vi "writeBits.vi"(0 "I2C Ref Out":T3, 5 "Params":T2={"length"=0, "bitStart"=0, "data"=0, "Register Addresses"=107} {"Register Addresses" items=["SELF_TEST_X"=13, "SELF_TEST_Y"=14, "SELF_TEST_Z"=15, "SELF_TEST_A"=16, "SMPLRT_DIV"=25, "CONFIG"=26, "GYRO_CONFIG"=27, "ACCEL_CONFIG"=28, "MOT_THR"=31, "FIFO_EN"=35, "I2C_MST_CTRL"=36, "I2C_SLV0_ADDR"=37, "I2C_SLV0_REG"=38, "I2C_SLV0_CTRL"=39, "I2C_SLV1_ADDR"=40, "I2C_SLV1_REG"=41, "I2C_SLV1_CTRL"=42, "I2C_SLV2_ADDR"=43, "I2C_SLV2_REG"=44, "I2C_SLV2_CTRL"=45, "I2C_SLV3_ADDR"=46, "I2C_SLV3_REG"=47, "I2C_SLV3_CTRL"=48, "I2C_SLV4_ADDR"=49, "I2C_SLV4_REG"=50, "I2C_SLV4_DO"=51, "I2C_SLV4_CTRL"=52, "I2C_SLV4_DI"=53, "I2C_MST_STATUS"=54, "INT_PIN_CFG"=55, "INT_ENABLE"=56, "INT_STATUS"=58, "ACCEL_XOUT_H"=59, "ACCEL_XOUT_L"=60, "ACCEL_YOUT_H"=61, "ACCEL_YOUT_L"=62, "ACCEL_ZOUT_H"=63, "ACCEL_ZOUT_L"=64, "TEMP_OUT_H"=65, "TEMP_OUT_L"=66, "GYRO_XOUT_H"=67, "GYRO_XOUT_L"=68, "GYRO_YOUT_H"=69, "GYRO_YOUT_L"=70, "GYRO_ZOUT_H"=71, "GYRO_ZOUT_L"=72, "EXT_SENS_DATA_00"=73, "EXT_SENS_DATA_01"=74, "EXT_SENS_DATA_02"=75, "EXT_SENS_DATA_03"=76, "EXT_SENS_DATA_04"=77, "EXT_SENS_DATA_05"=78, "EXT_SENS_DATA_06"=79, "EXT_SENS_DATA_07"=80, "EXT_SENS_DATA_08"=81, "EXT_SENS_DATA_09"=82, "EXT_SENS_DATA_10"=83, "EXT_SENS_DATA_11"=84, "EXT_SENS_DATA_12"=85, "EXT_SENS_DATA_13"=86, "EXT_SENS_DATA_14"=87, "EXT_SENS_DATA_15"=88, "EXT_SENS_DATA_16"=89, "EXT_SENS_DATA_17"=90, "EXT_SENS_DATA_18"=91, "EXT_SENS_DATA_19"=92, "EXT_SENS_DATA_20"=93, "EXT_SENS_DATA_21"=94, "EXT_SENS_DATA_22"=95, "EXT_SENS_DATA_23"=96, "I2C_SLV0_DO"=99, "I2C_SLV1_DO"=100, "I2C_SLV2_DO"=101, "I2C_SLV3_DO"=102, "I2C_MST_DELAY_CTRL"=103, "SIGNAL_PATH_RESET"=104, "MOT_DETECT_CTRL"=105, "USER_CTRL"=106, "PWR_MGMT_1"=107, "PWR_MGMT_2"=108, "FIFO_COUNTH"=114, "FIFO_COUNTL"=115, "FIFO_R_W"=116, "WHO_AM_I"=117]}, 11 "error in (no error)":errorcluster) -> (4 "I2C Ref Out 2":T3={"myRIO Reference"={"myRIO Model"=enum."Unknown", "myRIO Hardware Reference"={"Generic FPGA Reference"=refnum, "Allow multiple opens"=FALSE}}, "I2C Channels Enum"=enum."Not Connected", "I2C Configuration"={"I2C Transfer Rate"=enum."Fast mode (400 kbps)"}}, 15 "error out":errorcluster)   [LabVIEW 2016]
uses:
  <vilib>/myRIO/Instrument Drivers/Onboard IO/I2C/typedefs/I2C Reference.ctl
  <vilib>/myRIO/Common/Instrument Driver Framework/Utilities/typedefs/myRIO Generic Hardware Reference.ctl
  <vilib>/myRIO/Common/Instrument Driver Framework/Utilities/typedefs/Hardware Version Enum.ctl
  <vilib>/myRIO/Common/Instrument Driver Framework/Utilities/typedefs/myRIO v1.0 Reference.ctl
  <vilib>/myRIO/Common/Instrument Driver Framework/Utilities/typedefs/Generic FPGA Reference.ctl
  <vilib>/myRIO/Common/Instrument Driver Framework/myRIO v1.0/I2C/typedefs/I2C Channels Enum.ctl
  <vilib>/myRIO/Instrument Drivers/Onboard IO/I2C/typedefs/I2C Configuration.ctl
  <vilib>/myRIO/Instrument Drivers/Onboard IO/I2C/typedefs/I2C Transfer Rate.ctl
  LIFA MPU-60X0 LV9/RegisterAddresses.ctl
  LIFA MPU-60X0 LV9/DeviceAddresses.ctl
  <vilib>/myRIO/Common/Instrument Driver Framework/myRIO v1.0/I2C/vis/myRIO v1.0 Write I2C.vi
  <vilib>/myRIO/Common/Instrument Driver Framework/myRIO v1.0/I2C/vis/myRIO v1.0 Read I2C.vi
  <vilib>/myRIO/Common/Instrument Driver Framework/roboRIO v1.0/I2C/vis/roboRIO v1.0 Write I2C.vi
  <vilib>/myRIO/Common/Instrument Driver Framework/roboRIO v1.0/I2C/vis/roboRIO v1.0 Read I2C.vi
  <vilib>/Utility/error.llb/Error Cluster From Error Code.vi
  <vilib>/myRIO/Instrument Drivers/Onboard IO/I2C/I2C.lvlib
  LIFA MPU-60X0 LV9/LIFA MPU-60X0.lvlib
panel:
  out "x .or. y?":u8
  out "element":u8
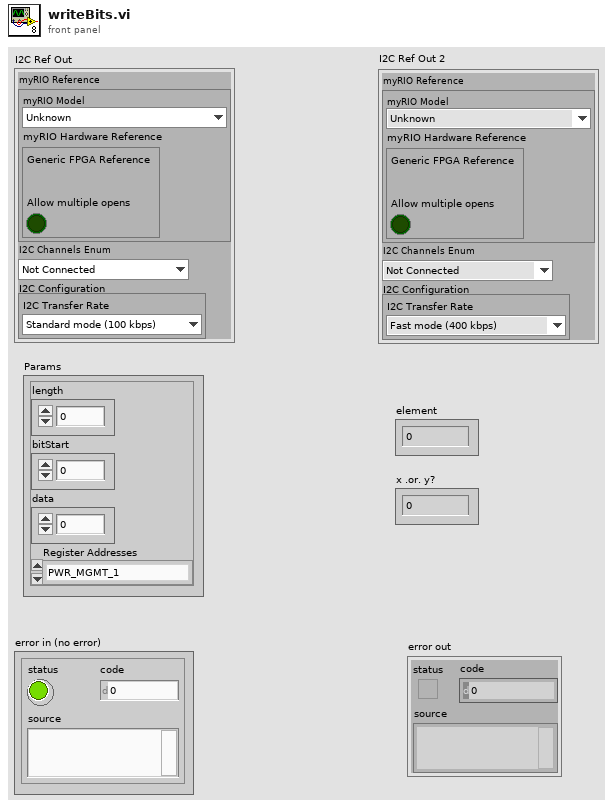
[diagram p1: front panel]
types:
  T1 = typedef "LIFA MPU-60X0.lvlib/RegisterAddresses.ctl" = u16
  T2 = cluster{"length":u8, "bitStart":u8, "data":u8, "Register Addresses":T1}
  T3 = typedef "I2C.lvlib/I2C Reference.ctl" = cluster{"myRIO Reference":T4, "I2C Channels Enum":T8, "I2C Configuration":T9}
  T4 = typedef "myRIO Generic Hardware Reference.ctl" = cluster{"myRIO Model":T5, "myRIO Hardware Reference":T6}
  T5 = typedef "Hardware Version Enum.ctl" = enum16{"Unknown", "myRIO-1900", "myRIO-1950", "roboRIO", "NI ELVIS RIO CM"}
  T6 = typedef "myRIO v1.0 Reference.ctl" = cluster{"Generic FPGA Reference":T7, "Allow multiple opens":bool}
  T7 = typedef "Generic FPGA Reference.ctl" = refnum<k20>
  T8 = typedef "I2C Channels Enum.ctl" = enum16{"Not Connected", "A/I2C", "B/I2C", "I2C/I2C"}
  T9 = typedef "I2C.lvlib/I2C Configuration.ctl" = cluster{"I2C Transfer Rate":T10}
  T10 = typedef "I2C.lvlib/I2C Transfer Rate.ctl" = enum16{"Standard mode (100 kbps)", "Fast mode (400 kbps)"}
  T11 = typedef "LIFA MPU-60X0.lvlib/DeviceAddresses.ctl" = u8
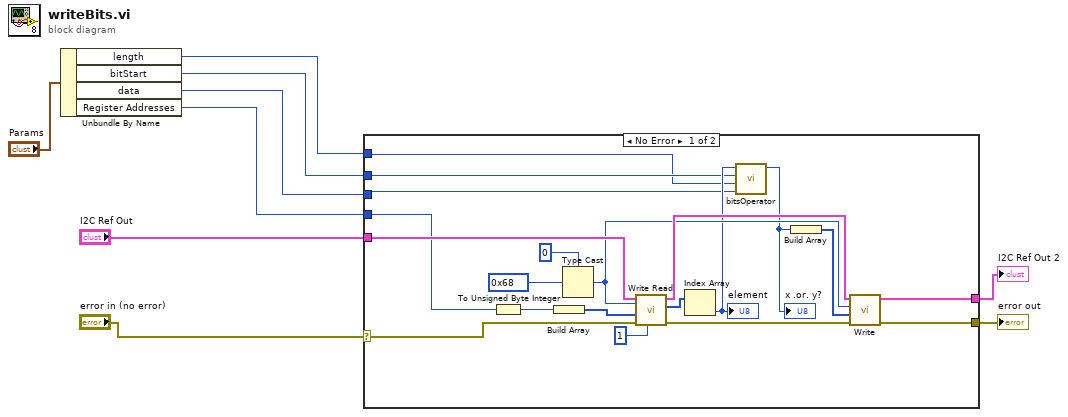
[diagram p0: block diagram]
diagram:
  n1 = Unbundle By Name("Params") -> ("length"=w3:u8, "bitStart"=w4:u8, "data"=w2:u8, "Register Addresses"=w1:T1)
  n2 = case shown="No Error" "error in (no error)" {
    selector: "error in (no error)" -> [w15 w30]
    tunnel: "I2C Ref Out" -> [w24 w31]
    tunnel: [w17 w31] -> w8
    tunnel: [w16 w30] -> w7
    tunnel: w4 -> [w13 _]
    tunnel: w3 -> [w12 _]
    tunnel: w2 -> [w11 _]
    tunnel: w1 -> [w10 _]
    frame No Error {
      w28 = T11 104 items=["0x68"=104, "0x69"=105] ("Device Address")
      n3 = To Unsigned Byte Integer(number=w10) -> (unsigned 8bit integer=w21:u8)
      n4 = Build Array(w21) -> (w29:u8[])
      n5 = Type Cast(type=u8 0 ("Slave Address (7-bit)"), x=w28) -> (*(type *) &x=w23:u8)
      n6 = call <vilib>:"Write Read.vi"("Byte Count"=u32 1, "error in (no error)"=w15, "Bytes to Write"=w29, "Slave Address (7-bit)"=w23, "I2C Ref In"=w24) -> ("error out"=w26:errorcluster, "Bytes Read"=w27:u8[], "I2C Ref Out"=w25:T3)  [unwired: 3 in]
      n7 = Index Array(array=w27) -> (element=w20:u8)  [unwired: 1 in]
      "element" <- w20
      n8 = call "bitsOperator.vi"("b"=w20, "bitStart"=w13, "length"=w12, "data"=w11) -> ("x .or. y?"=w19:u8)  [unwired: 6 in]
      "x .or. y?" <- w19
      n9 = Build Array(w19) -> (w18:u8[])
      n10 = call <vilib>:"Write.vi"("error in (no error)"=w26, "Bytes to Write"=w18, "Slave Address (7-bit)"=w23, "I2C Ref In"=w25) -> ("error out"=w16:errorcluster, "I2C Ref Out"=w17:T3)  [unwired: 6 in]
    }
    frame Error {
    }
  }
  "I2C Ref Out 2" <- w8
  "error out" <- w7
